vi "Main.vi"(11 "Module Admin":refnum<class "Delacor_lib_QMH_Module Admin.lvclass">) -> ()   [LabVIEW 2020, in "Shutter.lvlib"]
doc: "This template is based off of the Queued Message Handler design pattern and the Queued Message Handler project template that ships with LabVIEW.\n\nThe main difference is that the queue is private to this module and communication between modules is performed via Broadcast and Request events.\n\nRequest events are wrapped in public API methods and are handled in the Event Handling Loop (EHL) of this VI. Any module can register for Broadcast events sent by this module. The EHL generates messages based on user interface actions.\n\nThe Message Handling Loop (MHL) processes messages generated by the EHL, or by other messages. The messages are string values, so new messages can be added easily to the Message Cases case structure in the MHL. Each message cluster can also provide an optional value for Message Data, which is a variant that can be converted to whatever message-specific data is required.\n_____\nBased on Delacor QMH Project Template 5.0.0.82."
uses:
  Shutter.lvlib
  <vilib>/Delacor/Delacor QMH/Libraries/Module Admin_class/Delacor_lib_QMH_Module Admin.lvclass
  Module Data--cluster.ctl
  Shutter State.ctl
  Stop Argument--cluster.ctl
  <vilib>/Delacor/Delacor QMH/Libraries/Message Queue_class/Delacor_lib_QMH_Message Queue.lvclass/Delacor_lib_QMH_Message Queue.ctl
  <vilib>/Delacor/Delacor QMH/Libraries/Module Admin_class/Delacor_lib_QMH_Module Admin.lvclass/Delacor_lib_QMH_Module Admin.ctl
  Set Shutter State Argument--cluster.ctl
  Set Shutter State (Reply Payload)--cluster.ctl
  Get Shutter State Argument--cluster.ctl
  Get Shutter State (Reply Payload)--cluster.ctl
  <vilib>/Utility/miscctls.llb/LVPointTypeDef.ctl
  <vilib>/Delacor/Delacor QMH/Libraries/Message Queue_class/Delacor_lib_QMH_Enqueue Message (Single).vi
  <vilib>/Delacor/Delacor QMH/Libraries/Module Admin_class/Delacor_lib_QMH_Get External Launch.vi
  <vilib>/Utility/error.llb/Error Cluster From Error Code.vi
  <vilib>/ErrorRing/Error Ring.xnode
  <vilib>/Delacor/Delacor QMH/Libraries/Message Queue_class/Delacor_lib_QMH_Message Queue.lvclass
panel:
  in  "Close Shutter":bool
  in  "Open Shutter":bool
  out "Shutter":bool
  in  "Serial Number":i32
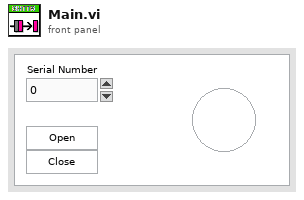
[diagram p1: front panel]
types:
  T1 = typedef "Shutter.lvlib/Request Events--cluster.ctl" = cluster{"Stop Module":refnum<user-event>, "Show Panel":refnum<user-event>, "Hide Panel":refnum<user-event>, "Get Module Execution Status":refnum<user-event>, "Show Diagram":refnum<user-event>, "Set Shutter State":refnum<user-event>, "Get Shutter State":refnum<user-event>}
  T2 = typedef "Shutter.lvlib/Module Data--cluster.ctl" = cluster{"Status":string, "Reference":refnum<k7>, "plState":i32}
  T3 = typedef "Shutter State.ctl" = enum16{"None", "Open", "Closed"}
  T4 = enum32{"invalid lock state", "Not Locked", "Locked (No Password)", "Password-protected"}
  T5 = typedef "Shutter.lvlib/Stop Argument--cluster.ctl" = cluster{"Origin":string, "Exit via Stop Module Req?":bool, "Wait for Module to stop?":bool}
  T6 = typedef "Shutter.lvlib/Set Shutter State Argument--cluster.ctl" = cluster{"Shutter State":T3, "Wait Notifier":refnum<notifier>, "wait for reply":bool}
  T7 = typedef "Shutter.lvlib/Get Shutter State Argument--cluster.ctl" = cluster{"Wait Notifier":refnum<notifier>, "wait for reply":bool}
  T8 = typedef "LVPointTypeDef.ctl" = cluster{"Horizontal":i16, "Vertical":i16}
  T9 = enum32{"Invalid", "Standard", "Closed", "Hidden", "Minimized", "Maximized"}
  T10 = typedef "Shutter.lvlib/Set Shutter State (Reply Payload)--cluster.ctl" = cluster{"Shutter State":T3, "Set Shutter State_error":errorcluster}
  T11 = typedef "Shutter.lvlib/Get Shutter State (Reply Payload)--cluster.ctl" = cluster{"Shutter State":T3, "Get Shutter State_error":errorcluster}
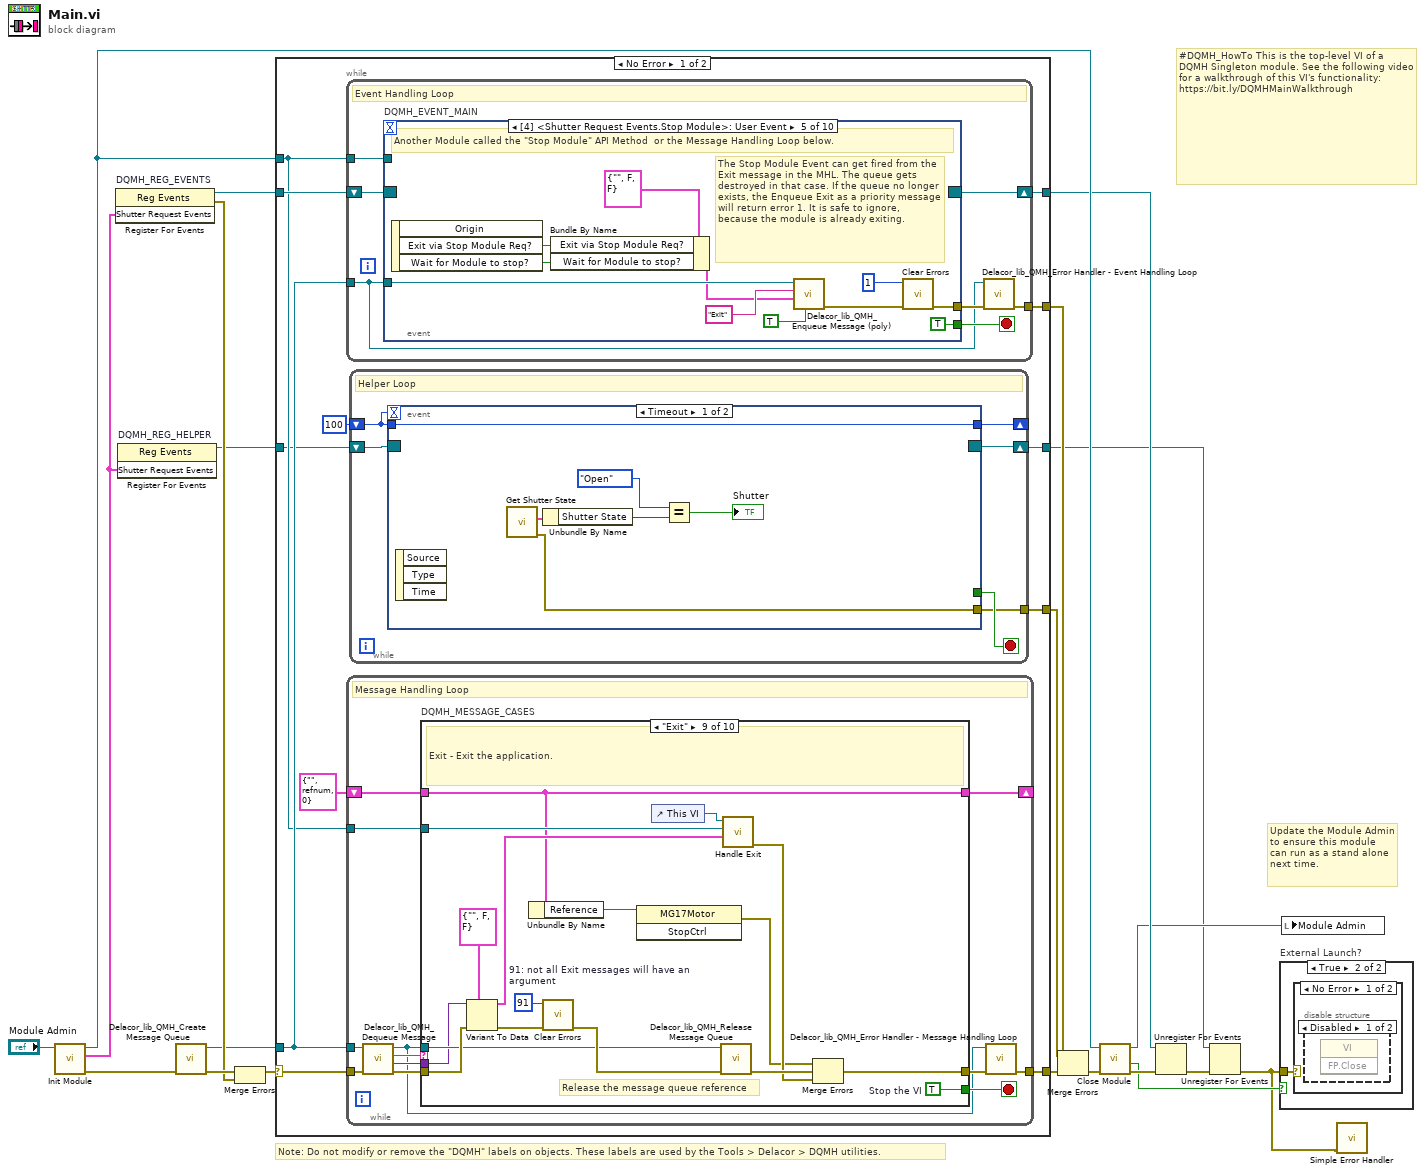
[diagram p0: block diagram]
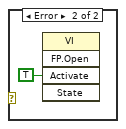
[diagram p4: hidden frame]
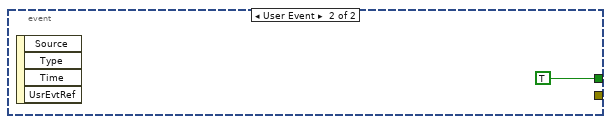
[diagram p5: hidden frame]
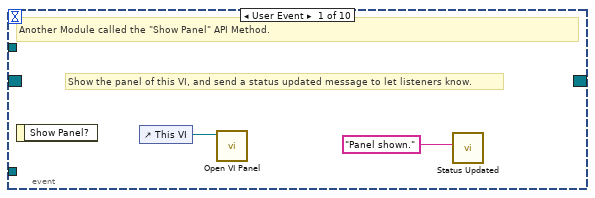
[diagram p6: hidden frame]
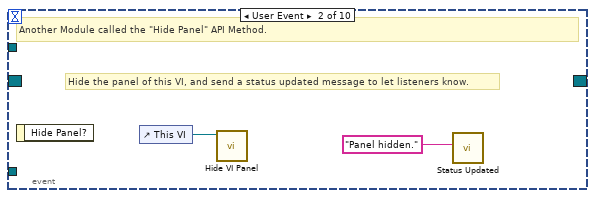
[diagram p7: hidden frame]
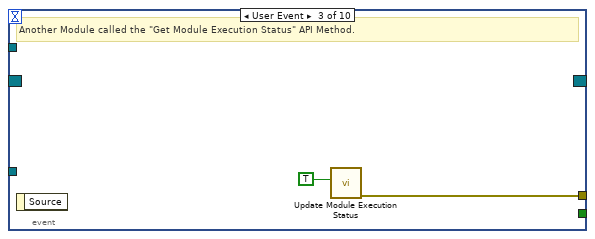
[diagram p8: hidden frame]
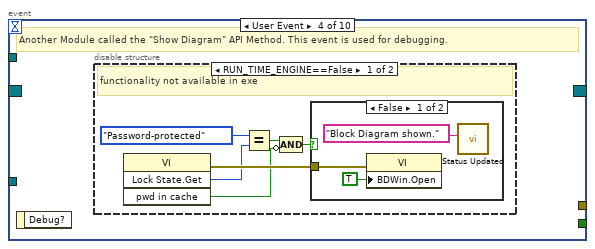
[diagram p9: hidden frame]
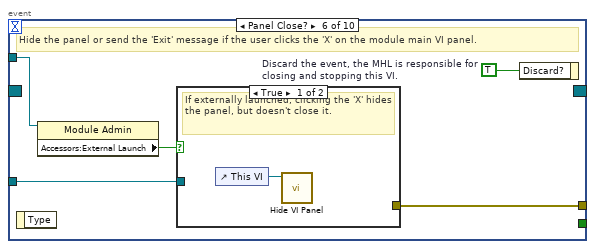
[diagram p12: hidden frame]
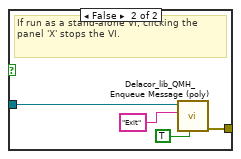
[diagram p13: hidden frame]
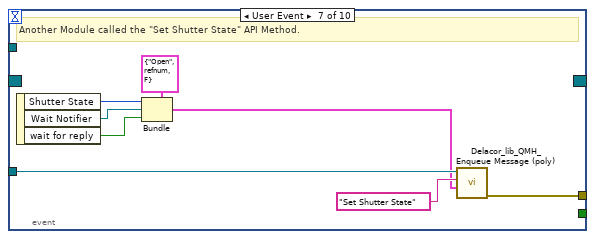
[diagram p14: hidden frame]
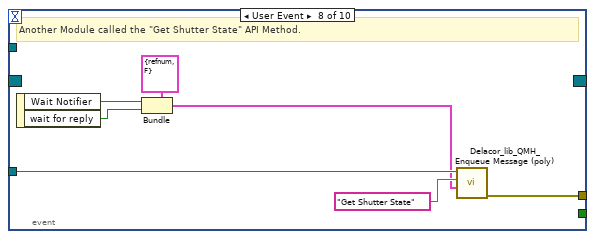
[diagram p15: hidden frame]
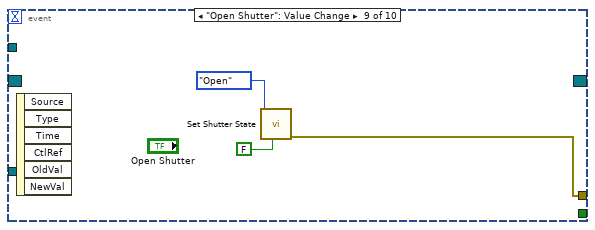
[diagram p16: hidden frame]
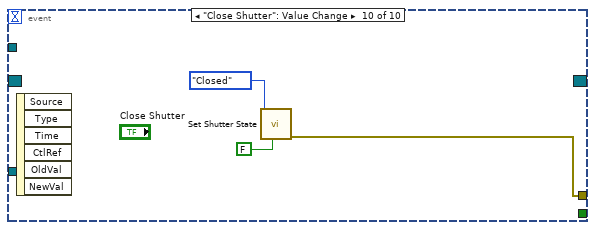
[diagram p17: hidden frame]
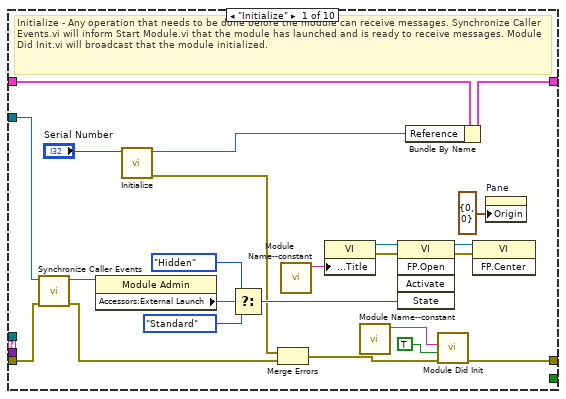
[diagram p18: hidden frame]
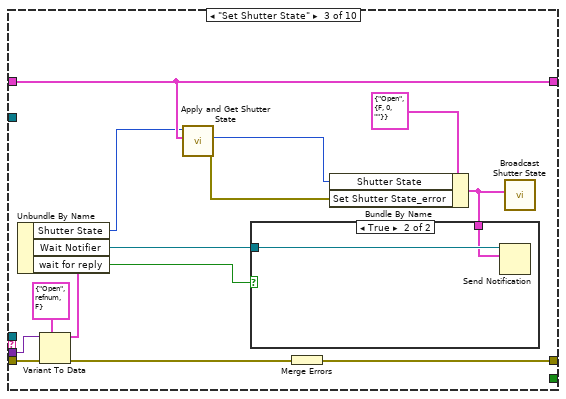
[diagram p20: hidden frame]
diagram:
  # "#DQMH_HowTo This is the top-level VI of a DQMH Singleton module. See the following video for a walkthrough of this VI's functionality: https://bit.ly/DQMHMainWalkthrough"
  # "Note: Do not modify or remove the \"DQMH\" labels on objects. These labels are used by the Tools > Delacor > DQMH utilities."
  # "Update the Module Admin to ensure this module can run as a stand alone next time."
  n1 = call "Init Module.vi"("Singleton Module Admin in"="Module Admin") -> ("error out"=w20:errorcluster, "Shutter Request Events"=w5:T1, "Singleton Module Admin out"=w12:refnum<class "Delacor_lib_QMH_Module Admin.lvclass">)  [unwired: 8 in]
  n2 = register-events "DQMH_REG_EVENTS"(w5) -> (reference out=w10:refnum<event-registration>, error out=w13:errorcluster)  [unwired: 2 in]
  n3 = register-events "DQMH_REG_HELPER"(w5) -> (reference out=w4:refnum<event-registration>)  [unwired: 2 in, 1 out]
  n4 = call <vilib>:"Delacor_lib_QMH_Create Message Queue.vi"("error in (no error)"=w20) -> ("error out"=w15:errorcluster, "Message Queue"=w9:refnum<class "Delacor_lib_QMH_Message Queue.lvclass">)  [unwired: 9 in]
  n5 = Merge Errors(w15, w13) -> (w14:errorcluster)
  n6 = case shown="No Error" w14 {
    selector: w14 -> [w31 w251]
    tunnel: [w33 w250] -> w21
    tunnel: [w30 w256] -> w11
    tunnel: w10 -> [w28 w256]
    tunnel: w9 -> [w27 w249]
    tunnel: [w32 _] -> w18
    tunnel: w12 -> [w26 w252]
    tunnel: w4 -> [w24 w248]
    tunnel: [w23 w248] -> w3
    tunnel: [w22 _] -> w2
    frame No Error {
      n7 = while {
        tunnel: w27 -> [w47]
        shift-right: [w50] -> w30
        shift-left: w28 -> [w51]
        tunnel: [w52] -> w32
        tunnel: w26 -> [w48]
        stop <- w49 stop-if-true
        # "Event Handling Loop"
        n8 = event "DQMH_EVENT_MAIN" shown="[4] <Shutter Request Events.Stop Module>: User Event" {
          selector: w51 -> [_ _ _ _ _ _ _ _ _ _]
          dyn-events: [_ _ _ _ _ _ _ _ _ _] -> w50
          timeout: _ -> [_ _ _ _ _ _ _ _ _ _]
          tunnel: [_ _ _ _ TRUE ("Discard?") _ _ _ _ _] -> w49
          tunnel: w47 -> [_ _ _ _ w75 w82 w97 w104 _ _]
          tunnel: [_ _ w59 _ w78 w84 w90 w98 w106 w109] -> w53
          tunnel: w48 -> [_ _ _ _ _ w81 _ _ _ _]
          event User Event {
            # "Show the panel of this VI, and send a status updated message to let listeners know."
            # "Another Module called the \"Show Panel\" API Method."
            n9 = event-data() -> ()  [unwired: 1 in, 1 out]
            n10 = control-ref of="This VI"() -> (w55:refnum<vi>)
            n11 = call "Open VI Panel.vi"("VI"=w55) -> ()  [unwired: 10 in, 1 out]
            n12 = call "Status Updated.vi"("Status"="Panel shown." ("format string")) -> ()  [unwired: 10 in, 1 out]
          }
          event User Event {
            # "Hide the panel of this VI, and send a status updated message to let listeners know."
            # "Another Module called the \"Hide Panel\" API Method."
            n13 = event-data() -> ()  [unwired: 1 in, 1 out]
            n14 = control-ref of="This VI"() -> (w57:refnum<vi>)
            n15 = call "Hide VI Panel.vi"("VI"=w57) -> ()  [unwired: 10 in, 1 out]
            n16 = call "Status Updated.vi"("Status"="Panel hidden." ("format string")) -> ()  [unwired: 10 in, 1 out]
          }
          event User Event {
            # "Another Module called the \"Get Module Execution Status\" API Method."
            n17 = event-data() -> ()  [unwired: 1 in, 1 out]
            n18 = call "Update Module Execution Status.vi"("Running?"=TRUE) -> ("error out"=w59:errorcluster)  [unwired: 10 in]
          }
          event User Event {
            # "Another Module called the \"Show Diagram\" API Method. This event is used for debugging."
            n19 = event-data() -> ()  [unwired: 1 in, 1 out]
            n20 = disable-structure shown="RUN_TIME_ENGINE==False" {
              frame condition #0 (active) {
                # "functionality not available in exe"
                n21 = invoke class="VI" method="Lock State.Get"() -> (error out=w65:errorcluster, "Get Lock State"=w64:T4, "pwd in cache"=w61:bool)  [unwired: 4 in, 1 out]
                n22 = Equal?(x=T4."Password-protected", y=w64) -> (x = y?=w62:bool)
                n23 = Compound Arithmetic op=AND(w62, invert w61) -> (w60:bool)
                n24 = case shown="False" w60 {
                  tunnel: w65 -> [w68 _]
                  frame False {
                    n25 = property class="VI"(error in=w68, "BDWin.Open"=TRUE ("Block Diagram Window:Open")) -> ()  [unwired: 1 in, 2 out]
                    n26 = call "Status Updated.vi"("Status"="Block Diagram shown." ("format string")) -> ()  [unwired: 10 in, 1 out]
                  }
                  frame True {
                    # "Password-protected VI, and the password is not in the cache. Do not show the diagram."
                  }
                }
              }
              frame condition #1 {
              }
            }
          }
          event User Event {
            # "The Stop Module Event can get fired from the Exit message in the MHL. The queue gets destroyed in that case. If the queue no longer exists, the Enqueue Exit as a priority message will return error 1. It is safe to ignore, because the module is already exiting."
            # "Another Module called the \"Stop Module\" API Method  or the Message Handling Loop below."
            n27 = event-data() -> ("Exit via Stop Module Req?"=w71:bool, "Wait for Module to stop?"=w70:bool)  [unwired: 1 in, 1 out]
            n28 = Bundle By Name(cluster=T5 {"Origin"="", "Exit via Stop Module Req?"=FALSE, "Wait for Module to stop?"=FALSE} ("Stop Argument"), "Exit via Stop Module Req?"=w71, "Wait for Module to stop?"=w70) -> (w69:T5)
            n29 = call-poly <vilib>:"Delacor_lib_QMH_Enqueue Message (poly).vi"("Priority Message? (F)"=TRUE, "Message Data"=w69, "Message"="Exit", "Message Queue in"=w75) -> ("error out"=w79:errorcluster)  [unwired: 6 in, 1 out]
            n30 = call <vilib>:"Clear Errors.vi"("error in (no error)"=w79, "specific error code to clear (0: all)"=1) -> ("error out"=w78:errorcluster)  [unwired: 4 in, 1 out]
          }
          event Panel Close? {
            w83 = TRUE  # Discard the event, the MHL is responsible for closing and stopping this VI.
            # "Hide the panel or send the 'Exit' message if the user clicks the 'X' on the module main VI panel."
            n31 = event-data() -> ()  [unwired: 1 in, 1 out]
            n32 = property class="Module Admin"(reference=w81) -> ("Accessors:External Launch"=w80:bool)  [unwired: 1 in, 2 out]
            n33 = case shown="True" w80 {
              tunnel: w82 -> [_ w88]
              tunnel: [_ w89] -> w84
              frame True {
                # "If externally launched, clicking the 'X' hides the panel, but doesn't close it."
                n34 = control-ref of="This VI"() -> (w85:refnum<vi>)
                n35 = call "Hide VI Panel.vi"("VI"=w85) -> ()  [unwired: 10 in, 1 out]
              }
              frame False {
                # "If run as a stand-alone VI, clicking the panel 'X' stops the VI."
                n36 = call-poly <vilib>:"Delacor_lib_QMH_Enqueue Message (poly).vi"("Priority Message? (F)"=TRUE, "Message"="Exit", "Message Queue in"=w88) -> ("error out"=w89:errorcluster)  [unwired: 7 in, 1 out]
              }
            }
            n37 = event-data("Discard?"=w83) -> ()  [unwired: 1 in, 1 out]
          }
          event User Event {
            # "Another Module called the \"Set Shutter State\" API Method."
            n38 = event-data() -> ("Shutter State"=w93:T3, "Wait Notifier"=w92:refnum<notifier>, "wait for reply"=w91:bool)  [unwired: 1 in]
            n39 = Bundle(cluster=T6 {"Shutter State"=enum."Open", "Wait Notifier"=refnum, "wait for reply"=FALSE} ("Set Shutter State Argument"), "Shutter State"=w93, "Wait Notifier"=w92, "wait for reply"=w91) -> (w94:T6)
            n40 = call-poly <vilib>:"Delacor_lib_QMH_Enqueue Message (poly).vi"("Message Data"=w94, "Message"="Set Shutter State", "Message Queue in"=w97) -> ("error out"=w90:errorcluster)  [unwired: 7 in, 1 out]
          }
          event User Event {
            # "Another Module called the \"Get Shutter State\" API Method."
            n41 = event-data() -> ("Wait Notifier"=w100:refnum<notifier>, "wait for reply"=w99:bool)  [unwired: 1 in]
            n42 = Bundle(cluster=T7 {"Wait Notifier"=refnum, "wait for reply"=FALSE} ("Get Shutter State Argument"), "Wait Notifier"=w100, "wait for reply"=w99) -> (w101:T7)
            n43 = call-poly <vilib>:"Delacor_lib_QMH_Enqueue Message (poly).vi"("Message Data"=w101, "Message"="Get Shutter State", "Message Queue in"=w104) -> ("error out"=w98:errorcluster)  [unwired: 7 in, 1 out]
          }
          event "Open Shutter": Value Change {
            n44 = event-data() -> ()  [unwired: 1 in, 6 out]
            n45 = call "Set Shutter State.vi"("wait for reply (T)"=FALSE, "Shutter State"=Shutter_State."Open") -> ("error out"=w106:errorcluster)  [unwired: 7 in, 2 out]
          }
          event "Close Shutter": Value Change {
            n46 = event-data() -> ()  [unwired: 1 in, 6 out]
            n47 = call "Set Shutter State.vi"("wait for reply (T)"=FALSE, "Shutter State"=Shutter_State."Closed") -> ("error out"=w109:errorcluster)  [unwired: 7 in, 2 out]
          }
        }
        n48 = call-dynamic "Delacor_lib_QMH_Error Handler - Event Handling Loop.vi"("error in (no error)"=w53, "Message Queue in"=w47) -> ("dup error in"=w52:errorcluster)  [unwired: 8 in, 1 out]
      }
      n49 = while {
        tunnel: w27 -> [w113]
        shift-right: [w117] -> _
        shift-left: T2 {"Status"="", "Reference"=refnum, "plState"=0} ("Data Cluster") -> [w118]
        tunnel: w31 -> [w121]
        tunnel: [w119] -> w33
        tunnel: w26 -> [w111]
        stop <- w116 stop-if-true
        # "Message Handling Loop"
        n50 = call-dynamic "Delacor_lib_QMH_Dequeue Message.vi"("error in (no error)"=w121, "Message Queue in"=w113) -> ("error out"=w120:errorcluster, "Message Data"=w114:variant, "Message"=w115:string, "Message Queue out"=w112:refnum<class "Delacor_lib_QMH_Message Queue.lvclass">)  [unwired: 6 in]
        n51 = case "DQMH_MESSAGE_CASES" shown="\"Exit\"" w115 {
          selector: w115 -> [_ _ _ _ _ _ _ _ _ w235]
          tunnel: w112 -> [_ _ _ _ _ _ _ w203 w227 _]
          tunnel: w120 -> [w143 w147 w161 w180 w185 w187 w192 w210 w233 w237]
          tunnel: [w141 w147 w152 w172 w184 w187 w191 w206 w230 w238] -> w122
          tunnel: w118 -> [w132 w146 w151 w171 w183 w186 w189 w205 w219 w236]
          tunnel: [w131 w146 w151 w167 w183 w186 w189 w205 w219 w236] -> w117
          tunnel: [_ _ _ _ _ _ _ _ w226 _] -> w116
          tunnel: w114 -> [_ _ w159 w178 _ _ _ w204 w225 _]
          tunnel: w111 -> [w133 _ _ _ _ _ _ w202 w220 _]
          frame "Initialize" {
            # "Initialize - Any operation that needs to be done before the module can receive messages. Synchronize Caller Events.vi will inform Start Module.vi that the module has launched and is ready to receive messages. Module Did Init.vi will broadcast that the module initialized."
            n52 = call "Synchronize Caller Events.vi"("error in (no error)"=w143, "Singleton Module Admin in"=w133) -> ("error out"=w142:errorcluster, "Singleton Module Admin out"=w128:refnum<class "Delacor_lib_QMH_Module Admin.lvclass">)  [unwired: 8 in]
            n53 = property class="Module Admin"(reference=w128) -> ("Accessors:External Launch"=w137:bool)  [unwired: 1 in, 2 out]
            n54 = call "Initialize.vi"("Serial Number"="Serial Number") -> ("error out"=w123:errorcluster, "reference out"=w125:refnum<k7>)  [unwired: 9 in]
            n55 = Select(t=T9."Hidden" ("State"), s=w137, f=T9."Standard" ("State")) -> (s? t:f=w134:T9)
            n56 = Merge Errors(w123, w142) -> (w124:errorcluster)
            n57 = call "Module Name--constant.vi"() -> ("Module Name"=w140:string)  [unwired: 11 in]
            n58 = property class="VI"("Front Panel.Title"=w140) -> (reference out=w139:refnum<vi>, error out=w145:errorcluster)  [unwired: 2 in]
            n59 = call "Module Name--constant.vi"() -> ("Module Name"=w129:string)  [unwired: 11 in]
            n60 = invoke class="VI" method="FP.Open"(reference=w139, error in=w145, "State"=w134) -> (reference out=w138:refnum<vi>, error out=w144:errorcluster)  [unwired: 2 in, 3 out]
            n61 = Bundle By Name(cluster=w132, "Reference"=w125) -> (w131:T2)
            n62 = call "Module Did Init.vi"("error in (no error)"=w124, "Initialized?"=TRUE, "Origin"=w129) -> ("error out"=w141:errorcluster)  [unwired: 8 in]
            n63 = invoke class="VI" method="FP.Center"(reference=w138, error in=w144) -> ()  [unwired: 1 in, 3 out]
            n64 = property on="Pane" class="Pane"("Origin"=T8 {"Horizontal"=0, "Vertical"=0}) -> ()  [unwired: 2 in, 2 out]
          }
          frame "--- Module Specific ---" {
            # "Separator -- The following cases handle messages specific to this Module."
          }
          frame "Set Shutter State" {
            n65 = Variant To Data(error in=w161, type=T6 {"Shutter State"=enum."Open", "Wait Notifier"=refnum, "wait for reply"=FALSE} ("Set Shutter State Argument"), Variant=w159) -> (data=w157:T6, error out=w160:errorcluster)
            n66 = Unbundle By Name(w157) -> ("Shutter State"=w150:T3, "Wait Notifier"=w156:refnum<notifier>, "wait for reply"=w155:bool)
            n67 = call "Apply and Get Shutter State.vi"("Data Cluster"=w151, "Shutter State"=w150) -> ("error out"=w149:errorcluster, "plState"=w148:i32)  [unwired: 7 in, 1 out]
            n68 = Merge Errors(w160) -> (w152:errorcluster)
            n69 = Bundle By Name(cluster=T10 {"Shutter State"=enum."Open", "Set Shutter State_error"={"status"=FALSE, "code"=0, "source"=""}} ("Set Shutter State (Reply Payload)"), "Shutter State"=w148, "Set Shutter State_error"=w149) -> (w154:T10)
            n70 = case shown="True" w155 {
              tunnel: w156 -> [_ w163]
              tunnel: w154 -> [_ w162]
              frame False {
              }
              frame True {
                n71 = Send Notification(notification=w162, notifier=w163) -> ()  [unwired: 1 in, 2 out]
              }
            }
            n72 = call "Broadcast Shutter State.vi"("Reply Payload"=w154) -> ()  [unwired: 10 in, 1 out]
          }
          frame "Get Shutter State" {
            n73 = Unbundle By Name(w171) -> ("Reference"=w170:refnum<k7>, "plState"=w168:i32)
            n74 = Variant To Data(error in=w180, type=T7 {"Wait Notifier"=refnum, "wait for reply"=FALSE} ("Get Shutter State Argument"), Variant=w178) -> (data=w176:T7, error out=w179:errorcluster)
            n75 = invoke class="MG17Motor" method="SC_GetOPState"(reference=w170, "lChanID"=0, "plState"=w168) -> (error out=w169:errorcluster, "plState"=w164:i32)  [unwired: 2 in, 3 out]
            n76 = Unbundle By Name(w176) -> ("Wait Notifier"=w175:refnum<notifier>, "wait for reply"=w174:bool)
            n77 = Bundle By Name(cluster=w171, "plState"=w164) -> (w167:T2)
            n78 = Merge Errors(w179, w169) -> (w172:errorcluster)
            n79 = Bundle By Name(cluster=T11 {"Shutter State"=enum."None", "Get Shutter State_error"={"status"=FALSE, "code"=0, "source"=""}} ("Get Shutter State (Reply Payload)"), "Shutter State"=w164, "Get Shutter State_error"=w169) -> (w166:T11)
            n80 = case shown="True" w174 {
              tunnel: w175 -> [_ w182]
              tunnel: w166 -> [_ w181]
              frame False {
              }
              frame True {
                n81 = Send Notification(notification=w181, notifier=w182) -> ()  [unwired: 1 in, 2 out]
              }
            }
            n82 = call "Broadcast Shutter State.vi"("Reply Payload"=w166) -> ()  [unwired: 10 in, 1 out]
          }
          frame "---Copy This Frame---" {
            # "Duplicate this frame when creating new messages.  Change this comment in the duplicated frame to describe this message."
            n83 = Merge Errors(w185) -> (w184:errorcluster)
          }
          frame "--- Exit and Error Handling---" {
            # "Separator - The following cases handle errors and exit messages."
          }
          frame "Simulate MHL Error" {
            # "#DQMH_HowTo The 'Simulate MHL Error' button  illustrates how the MHL handles errors. This event is instructional in nature and can be removed."
            # "Simulate an error occurring at the MHL"
            n84 = call "Module Name--constant.vi"() -> ("Module Name"=w188:string)  [unwired: 11 in]
            n85 = xnode "Error Ring"("parameter 0"=w188) -> ("error out"=w190:errorcluster)
            n86 = Merge Errors(w192, w190) -> (w191:errorcluster)
          }
          frame "Error" {
            # "#CodeRecommended - If you ever change the name of this \"Error\" message, you'll need to update the name in the Check Loop Error.vi as well."
            # "#CodeRecommended - If the module is running in standalone mode (External Launch = FALSE), this code will pop up an error dialog and call the 'Exit' message if an error occurs. Add more fine-grained error handling here."
            # "Error - Check the error message data and respond accordingly. This message is sent by the \"Error Handler\" VIs at the end of each loop in this application."
            n87 = property class="Module Admin"(reference=w202) -> ("Accessors:External Launch"=w201:bool)  [unwired: 1 in, 2 out]
            n88 = Variant To Data(error in=w210, type=errorcluster {"status"=FALSE, "code"=0, "source"=""} ("error constant"), Variant=w204) -> (data=w211:errorcluster, error out=w208:errorcluster)
            n89 = call "Module Name--constant.vi"() -> ("Module Name"=w200:string)  [unwired: 11 in]
            n90 = call "Error Reported.vi"("Additional Information"=w200, "Error"=w211) -> ()  [unwired: 9 in, 1 out]
            n91 = case shown="False" w201 {
              tunnel: [w216 _] -> w207
              tunnel: w203 -> [w214 _]
              tunnel: w211 -> [w215 _]
              frame False {
                # "If the module is running standalone, then pop up an error dialog and call the \"Exit\" message."
                n92 = call <vilib>:"Simple Error Handler.vi"("error in (no error)"=w215) -> ()  [unwired: 4 in, 5 out]
                n93 = call-poly <vilib>:"Delacor_lib_QMH_Enqueue Message (poly).vi"("Priority Message? (F)"=TRUE, "Message"="Exit", "Message Queue in"=w214) -> ("error out"=w216:errorcluster)  [unwired: 7 in, 1 out]
              }
              frame True {
                # "If the module was launched externally, calling the Error Reported broadcast VI is the only action performed by the \"Error\" message. The module's caller can then process the error appropriately."
              }
            }
            n94 = Merge Errors(w208, w207) -> (w206:errorcluster)
          }
          frame "Exit" {
            w224 = 91  # 91: not all Exit messages will have an argument
            w226 = TRUE  # Stop the VI
            # "Release the message queue reference"
            # "Exit - Exit the application."
            n95 = Variant To Data(error in=w233, type=T5 {"Origin"="", "Exit via Stop Module Req?"=FALSE, "Wait for Module to stop?"=FALSE} ("Stop Argument"), Variant=w225) -> (data=w222:T5, error out=w229:errorcluster)
            n96 = Unbundle By Name(w219) -> ("Reference"=w218:refnum<k7>)
            n97 = call <vilib>:"Clear Errors.vi"("error in (no error)"=w229, "specific error code to clear (0: all)"=w224) -> ("error out"=w232:errorcluster)  [unwired: 4 in, 1 out]
            n98 = invoke class="MG17Motor" method="StopCtrl"(reference=w218) -> (error out=w217:errorcluster)  [unwired: 2 in, 2 out]
            n99 = control-ref of="This VI"() -> (w221:refnum<vi>)
            n100 = call-dynamic "Delacor_lib_QMH_Release Message Queue.vi"("error in (no error)"=w232, "Message Queue"=w227) -> ("error out"=w231:errorcluster)  [unwired: 9 in]
            n101 = call "Handle Exit.vi"("Stop Argument"=w222, "Admin in"=w220, "VI reference"=w221) -> ("error out"=w228:errorcluster)  [unwired: 7 in, 1 out]
            n102 = Merge Errors(w217, w231, w228) -> (w230:errorcluster)
          }
          frame Default {
            # "'Default' case only runs if there is a message that isn't defined in any of the other cases.  Output a programming error."
            n103 = call "Module Name--constant.vi"() -> ("Module Name"=w234:string)  [unwired: 11 in]
            n104 = xnode "Error Ring"("parameter 0"=w235, "parameter 1"=w234) -> ("error out"=w239:errorcluster)
            n105 = Merge Errors(w237, w239) -> (w238:errorcluster)
          }
        }
        n106 = call-dynamic "Delacor_lib_QMH_Error Handler - Message Handling Loop.vi"("error in (no error)"=w122, "Message Queue in"=w112) -> ("dup error in"=w119:errorcluster)  [unwired: 8 in, 1 out]
      }
      n107 = while {
        shift-right: [w38] -> _
        shift-left: 100 -> [w39]
        shift-right: [w36] -> w23
        shift-left: w24 -> [w37]
        tunnel: [w34] -> w22
        stop <- w35 stop-if-true
        # "Helper Loop"
        n108 = event shown="[0] Timeout" {
          selector: w37 -> [_ _]
          dyn-events: [_ _] -> w36
          timeout: w39 -> [_ _]
          tunnel: w39 -> [w45 _]
          tunnel: [w45 _] -> w38
          tunnel: [_ TRUE] -> w35
          tunnel: [w44 _] -> w34
          event Timeout {
            n109 = event-data() -> ()  [unwired: 1 in, 3 out]
            n110 = call "Get Shutter State.vi"() -> ("error out"=w44:errorcluster, "Reply Payload"=w43:T11)  [unwired: 9 in, 1 out]
            n111 = Unbundle By Name(w43) -> ("Shutter State"=w42:T3)
            n112 = Equal?(x=Shutter_State."Open" ("Shutter State"), y=w42) -> (x = y?=→"Shutter":bool)
          }
          event User Event {
            n113 = event-data() -> ()  [unwired: 1 in, 4 out]
          }
        }
      }
    }
    frame Error {
      # "Synchronize Caller Events.vi will inform Start Module.vi that the module has launched and will let the code calling Start Module.vi register for broadcasts and would permit the caller receive the broadcast that an error occurred at launch time."
      n114 = call-dynamic "Delacor_lib_QMH_Release Message Queue.vi"("error in (no error)"=w251, "Message Queue"=w249) -> ("error out"=w250:errorcluster)  [unwired: 9 in]
      n115 = call "Synchronize Caller Events.vi"("Singleton Module Admin in"=w252) -> ("error out"=w257:errorcluster)  [unwired: 9 in, 1 out]
      n116 = call "Module Name--constant.vi"() -> ("Module Name"=w255:string)  [unwired: 11 in]
      n117 = Format Into String(format string="An error occurred during initialization. %s is no longer running.", w255) -> (resulting string=w253:string)  [unwired: 2 in, 1 out]
      n118 = Merge Errors(w250, w257) -> (w258:errorcluster)
      n119 = call "Error Reported.vi"("Additional Information"=w253, "Error"=w258) -> ()  [unwired: 9 in, 1 out]
    }
  }
  n120 = Merge Errors(w2, w18, w21) -> (w17:errorcluster)
  n121 = call "Close Module.vi"("error in (no error)"=w17, "Module Admin in"=w12) -> ("error out"=w19:errorcluster, "External Launch"=w6:bool, "Module Admin out"=w7:refnum<class "Delacor_lib_QMH_Module Admin.lvclass">)  [unwired: 7 in]
  n122 = Unregister For Events(event registration refnum=w11, error in=w19) -> (error out=w16:errorcluster)
  n123 = Unregister For Events(event registration refnum=w3, error in=w16) -> (error out=w1:errorcluster)
  n124 = case "External Launch?" shown="True" w6 {
    tunnel: w1 -> [_ w259]
    frame False {
    }
    frame True {
      n125 = case shown="No Error" w259 {
        frame No Error {
          n126 = disable-structure shown="Disabled" {
            frame Disabled {
              n127 = invoke class="VI" method="FP.Close"() -> ()  [unwired: 3 in, 3 out]
            }
            frame Enabled {
            }
          }
        }
        frame Error {
          n128 = invoke class="VI" method="FP.Open"("Activate"=TRUE ("Activate?")) -> ()  [unwired: 4 in, 5 out]
        }
      }
    }
  }
  n129 = local write "Module Admin"(w7) -> ()
  n130 = call <vilib>:"Simple Error Handler.vi"("error in (no error)"=w1) -> ()  [unwired: 4 in, 5 out]
